vi "User select_combobox.vi"(7 "조합?":bool=TRUE, 9 "문자열 입력":string, 11 "배열 입력":string[](array[string])) -> (3 "문자열 출력":string)   [LabVIEW 2020]
uses:
  Variables/Global_Cal Info.vi
panel:
  in  "기준기":string(combo) caption="기준기 선택/조합"
  in  "확인":bool
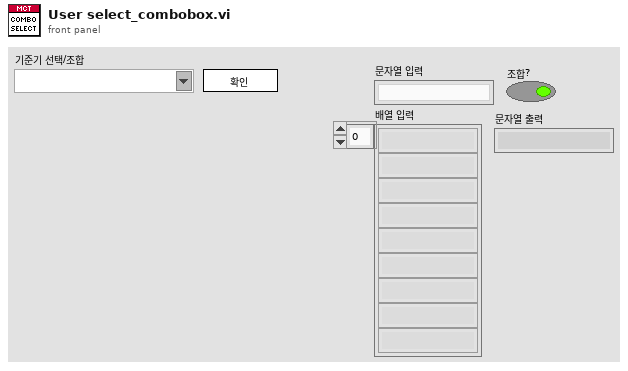
[diagram p1: front panel]
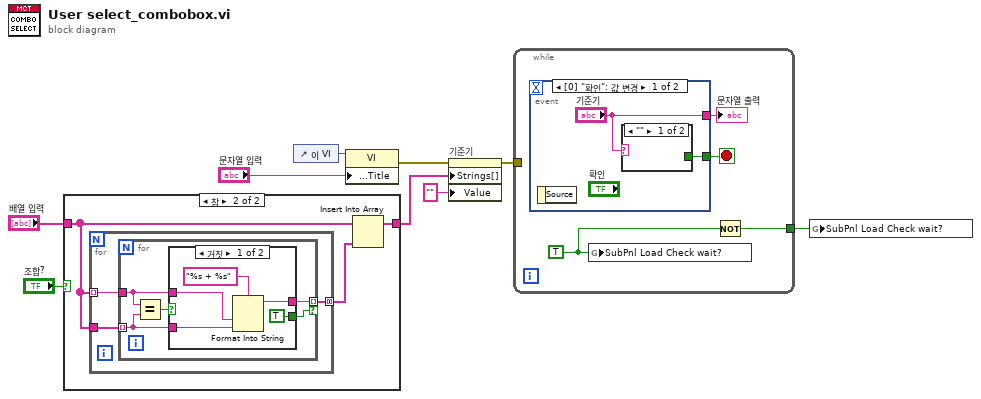
[diagram p0: block diagram]
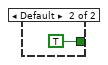
[diagram p4: hidden frame]
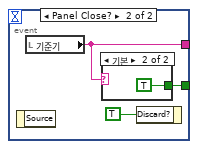
[diagram p5: hidden frame]
diagram:
  n1 = case shown="참" "조합?" {
    tunnel: "배열 입력" -> [w10 w13]
    tunnel: [w10 w11] -> w8
    frame False {
    }
    frame True {
      n2 = for {
        tunnel: w13 -> [w14] mode=indexing
        tunnel: w13 -> [w16]
        tunnel: [w15] -> w12 mode=concatenating
        n3 = for {
          tunnel: w16 -> [w20] mode=indexing
          tunnel: [w19] -> w15 mode=indexing if=w17
          tunnel: w14 -> [w21]
          n4 = Equal?(x=w21, y=w20) -> (x = y?=w18:bool)
          n5 = case shown="거짓" w18 {
            tunnel: w21 -> [w26 _]
            tunnel: w20 -> [w25 _]
            tunnel: [w24 _] -> w19
            tunnel: [TRUE _] -> w17
            frame False {
              n6 = Format Into String(format string="%s + %s" ("포맷 문자열"), w26, w25) -> (resulting string=w24:string)  [unwired: 2 in, 1 out]
            }
            frame True {
            }
          }
        }
      }
      n7 = Insert Into Array(array=w13, new element=w12) -> (w11:string[])  [unwired: 1 in]
    }
  }
  n8 = control-ref of="이 VI"() -> (w5:refnum<vi>)
  n9 = property class="VI"(reference=w5, "Front Panel.Title"="문자열 입력") -> (error out=w4:errorcluster)  [unwired: 1 in, 1 out]
  n10 = property on="기준기" class="CmbBox"(error in=w4, "Strings[]"=w8, "Value"="" ("기준기")) -> (error out=w7:errorcluster)  [unwired: 1 in, 1 out]
  n11 = while {
    tunnel: w7 -> [_]
    tunnel: [w27] -> w2
    stop <- w30 stop-if-true
    w28 = TRUE ("SubPnl Load Check wait?")
    n12 = event shown="[0] \"확인\": 값 변경" {
      selector: _ -> [_ _]
      dyn-events: _ -> [_ _]
      timeout: _ -> [_ _]
      tunnel: [w32 w35] -> w30
      tunnel: ["기준기" w34] -> w29
      event "확인": Value Change {
        n13 = event-data() -> ()  [unwired: 1 in, 1 out]
        n14 = case shown="\"\"" "기준기" {
          tunnel: [_ TRUE] -> w32
          frame "" {
          }
          frame Default {
          }
        }
      }
      event Panel Close? {
        n15 = event-data() -> ()  [unwired: 1 in, 1 out]
        n16 = local read "기준기"() -> (w34:string)
        n17 = case shown="기본" w34 {
          tunnel: [_ TRUE] -> w35
          frame "" {
          }
          frame Default {
          }
        }
        n18 = event-data("Discard?"=TRUE ("버림?")) -> ()  [unwired: 1 in, 1 out]
      }
    }
    "문자열 출력" <- w29
    n19 = global write "Global_Cal Info.vi" "SubPnl Load Check wait?"(w28) -> ()
    n20 = Not(x=w28) -> (.not. x?=w27:bool)
  }
  n21 = global write "Global_Cal Info.vi" "SubPnl Load Check wait?"(w2) -> ()
